vi "Get Behavior Flags.vi"(8 "error in (no error)":errorcluster, 11 "Element Array in":refnum<class "Element Array.lvclass">) -> (0 "error out":errorcluster, 2 "Behavior":T1={"Children"=enum."Multiple", "Editable"=FALSE, "XML uses />"=FALSE}, 3 "Element Array out":refnum<class "Element Array.lvclass">)   [LabVIEW 2023, in "VILab.lvlib" / "Element Array.lvclass"]
uses:
  Element Array.lvclass
  Data Item/Behavior Flags.ctl
  Data Item/Child Support.ctl
  Element Array.lvclass/Element Array.ctl
  Data Item/Data Item.lvclass
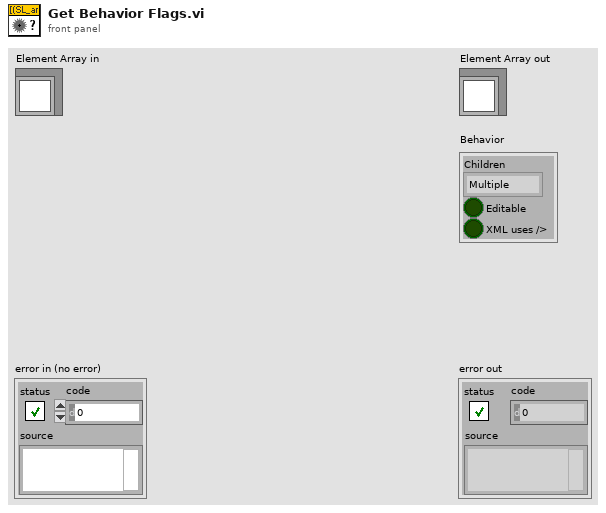
[diagram p1: front panel]
types:
  T1 = typedef "VILab.lvlib/Data Item.lvclass/Behavior Flags.ctl" = cluster{"Children":T2, "Editable":bool, "XML uses />":bool}
  T2 = typedef "VILab.lvlib/Data Item.lvclass/Child Support.ctl" = enum16{"None", "One", "At most one", "Multiple"}
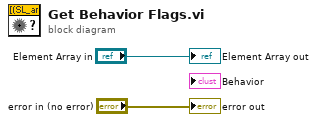
[diagram p0: block diagram]
diagram:
  "error out" <- "error in (no error)"
  "Element Array out" <- "Element Array in"
